vi "CRYAna TSR.vi"(0 "Response":dbl[](array[numeric]) format="%.2f", 1 "Abs/Rel":u16(ring) items=["Absolute", "Relative"], 2 "dz(Hz)":dbl=10.0, 3 "EQ information":T2={"Stimulus EQ Curve"={"Name"="", "Curve"=[], "X data"=1, "Y data"=1, "Z data"=1, "X axis"=0, "Y axis"=1, "Z axis"=1, "X unit"="Hz", "Y unit"="", "Z unit"="deg.", "X dB ref"=1.0, "Y dB ref"=1.0, "Z dB ref"=1.0, "single val"=FALSE, "protected"=FALSE, "display X"=TRUE, "display Y"=TRUE, "display Z"=TRUE, "Test Info"="", "Step No."=0, "Plot Settings"={"Color"=0, "Interpolation"=0, "Point Style"=0, "Line Style"=0, "Point Color"=0, "Line Width"=0, "Bar Plot Style"=0, "Fill To"=0}, "AutoProtect"=FALSE}, "EQ"=FALSE, "EQ Rate"=0.0} {"EQ Rate" format="%.2f"; "Stimulus EQ Curve"."Z data" items=["dB", "Lin"]; "Stimulus EQ Curve"."X data" items=["dB", "Lin"]; "Stimulus EQ Curve"."Y data" items=["dB", "Lin"]; "Stimulus EQ Curve"."Z dB ref" format="%.1f"; "Stimulus EQ Curve"."Z axis" items=["Log", "Lin"]; "Stimulus EQ Curve"."X dB ref" format="%.1f"; "Stimulus EQ Curve"."X axis" items=["Log", "Lin"]; "Stimulus EQ Curve"."Y axis" items=["Log", "Lin"]; "Stimulus EQ Curve"."Y dB ref" format="%.1f"; "Stimulus EQ Curve"."Curve"."z" format="%.2f"; "Stimulus EQ Curve"."Curve"."y" format="%.2f"; "Stimulus EQ Curve"."Curve"."x" format="%.2f"}, 5 "Harmonics":dbl[](array[numeric]) format="%.2f", 7 "Parameter In":T3 {"Over Sample Res" format="%.4f"; "Stop (ms)" format="%.4f"; "Start (ms)" format="%.4f"}, 9 "Resolution":u16=6, 11 "TSR params":T4 {"Sweep Time" format="%.2f"; "Amplit" format="%.2f"; "FStop" format="%.2f"; "FStart" format="%.2f"; "FSamp" format="%.2f"; "Tsamp" format="%.2f"; "NHarm" format="%.2f"; "MStart" format="%.2f"; "MStop" format="%.2f"; "NOffset" format="%.2f"}, 12 "Stimulus":dbl[](array[numeric]) format="%.2f", 15 "Impulse data type(db/Lin)":i32(ring) items=["dB", "Lin"]) -> (4 "Freq resp curves":cluster{cluster{"x":dbl, "y":dbl, "z":dbl}[]}[](array[cluster]) {"?"."z" format="%.2f"; "?"."y" format="%.2f"; "?"."x" format="%.2f"}, 8 "X axis, fundamental":dbl[](array[numeric]) format="%.2f", 10 "Total Noise":dbl[](array[numeric]), 13 "Impulse response":dbl[][](array[numeric]) format="%.2f", 14 "Impulse time axis":dbl[](array[numeric]) format="%.6f")   [LabVIEW 2013]
uses:
  Typedef Control/CRYData Cluster.ctl
  <vilib>/Analysis/NI_AALPro.lvlib
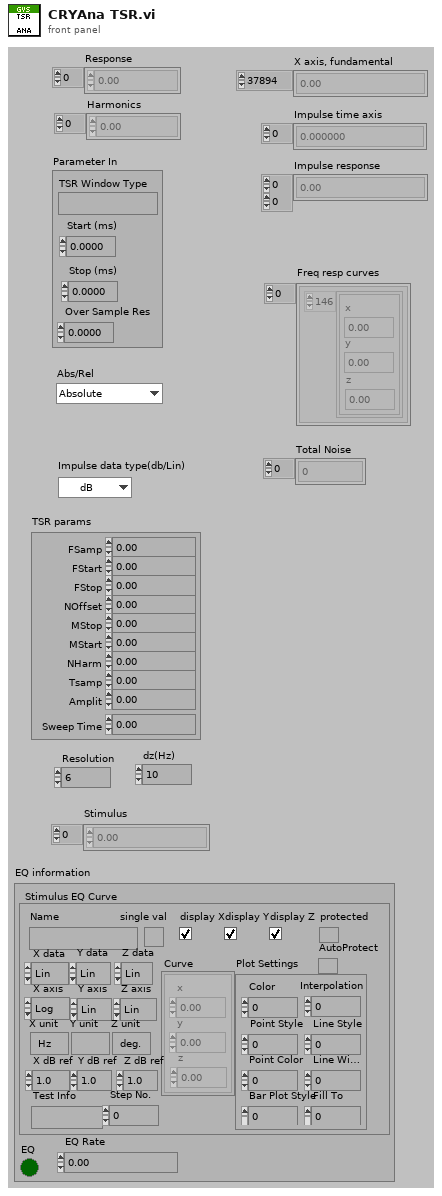
[diagram p1: front panel]
types:
  T1 = typedef "CRYData Cluster.ctl" = cluster{"Name":string, "Curve":cluster{"x":dbl, "y":dbl, "z":dbl}[], "X data":u16, "Y data":u16, "Z data":u16, "X axis":u16, "Y axis":u16, "Z axis":u16, "X unit":string, "Y unit":string, "Z unit":string, "X dB ref":dbl, "Y dB ref":dbl, "Z dB ref":dbl, "single val":bool, "protected":bool, "display X":bool, "display Y":bool, "display Z":bool, "Test Info":string, "Step No.":i32, "Plot Settings":cluster{"Color":u32, "Interpolation":u8, "Point Style":u8, "Line Style":u8, "Point Color":u32, "Line Width":u8, "Bar Plot Style":u8, "Fill To":i16}, "AutoProtect":bool}
  T2 = cluster{"Stimulus EQ Curve":T1, "EQ":bool, "EQ Rate":dbl}
  T3 = cluster{"TSR Window Type":string, "Start (ms)":dbl, "Stop (ms)":dbl, "Over Sample Res":dbl}
  T4 = cluster{"FSamp":dbl, "FStart":dbl, "FStop":dbl, "NOffset":dbl, "MStop":dbl, "MStart":dbl, "NHarm":dbl, "Tsamp":dbl, "Amplit":dbl, "Sweep Time":dbl}
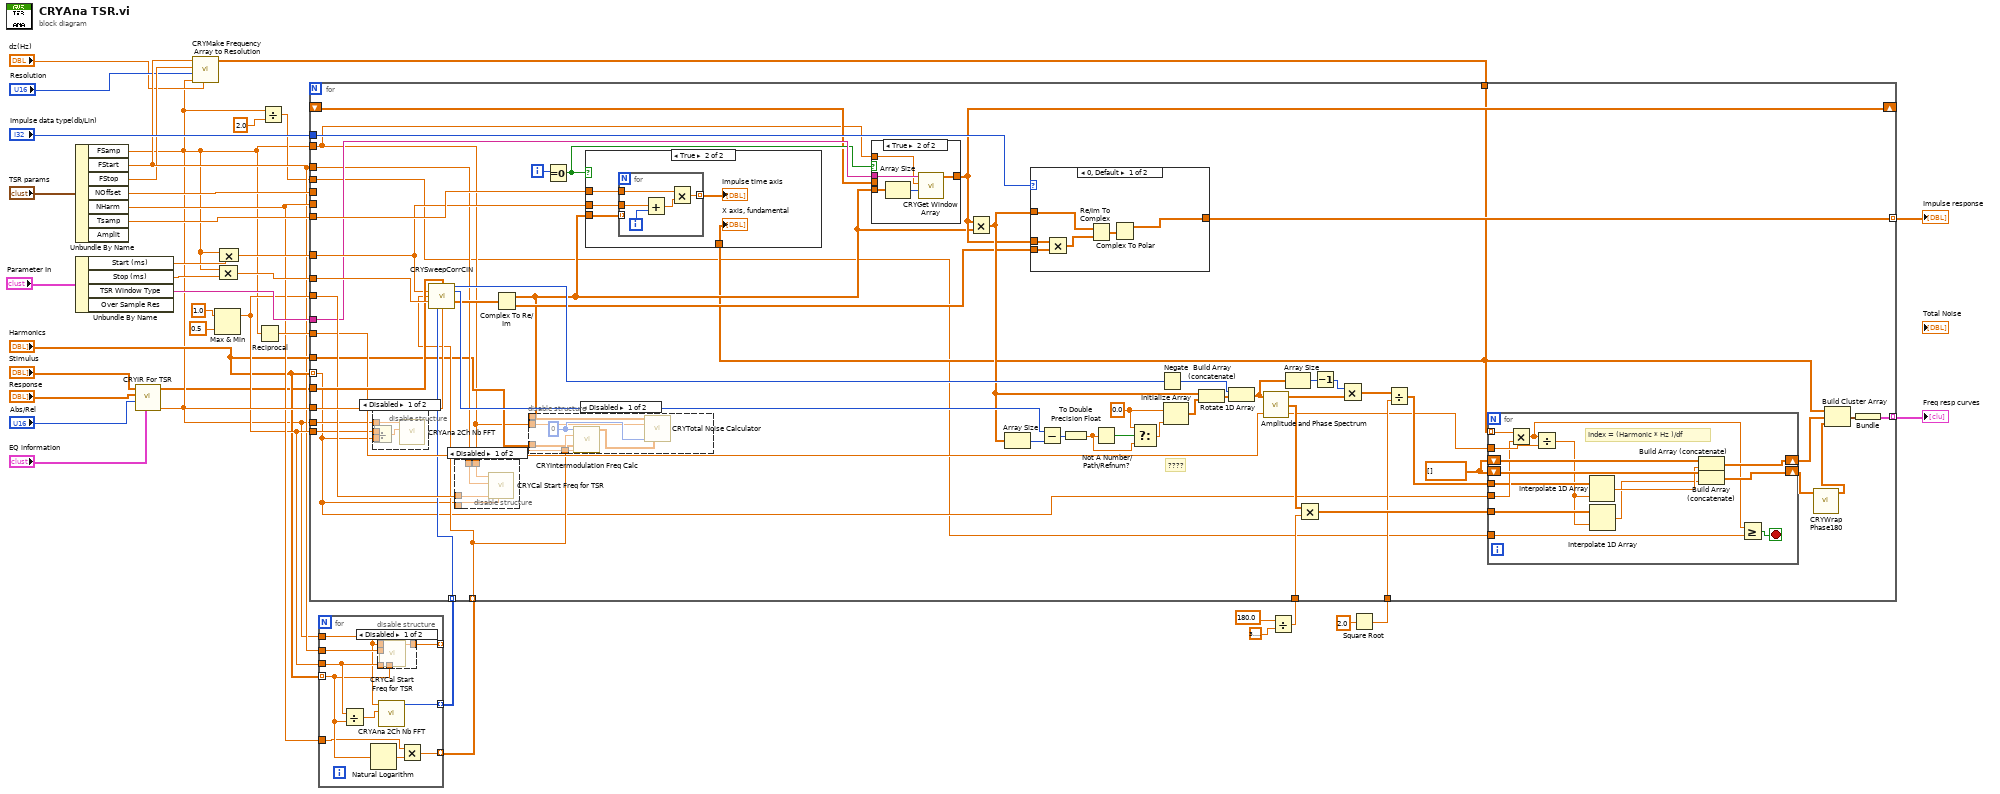
[diagram p0: block diagram]
diagram:
  n1 = Unbundle By Name("TSR params") -> ("FSamp"=w5:dbl, "FStart"=w12:dbl, "FStop"=w11:dbl, "NOffset"=w27:dbl, "NHarm"=w19:dbl, "Tsamp"=w39:dbl)  [unwired: 1 out]
  n2 = Unbundle By Name("Parameter In") -> ("Start (ms)"=w30:dbl, "Stop (ms)"=w29:dbl, "TSR Window Type"=w28:string)  [unwired: 1 out]
  n3 = call "CRYIR For TSR.vi"("EQ information"="EQ information", "Fs"=w5, "Abs/Rel"="Abs/Rel", "Response[y(t)]"="Response", "Stimulus[x(t)]"="Stimulus") -> ("T0"=w26:dbl, "Deconvolved Response"=w4:cdb[])  [unwired: 2 in, 3 out]
  n4 = call "CRYMake Frequency Array to Resolution.vi"("dz(Hz)"="dz(Hz)", "Fs"=w5, "Resolution"="Resolution", "Stop Freq"=w11, "Start Freq"=w12) -> ("Frequency Array"=w8:dbl[])  [unwired: 6 in]
  n5 = Max & Min(x=1.0, y=0.5) -> (max(x,y)=w14:dbl)  [unwired: 1 out]
  n6 = Compound Arithmetic op=MULTIPLY(w5, w29) -> (w33:dbl)
  n7 = Compound Arithmetic op=MULTIPLY(w5, w30) -> (w32:dbl)
  n8 = Reciprocal(x=w5) -> (1/x=w25:dbl)
  n9 = Divide(x=w5, y=2.0) -> (x/y=w6:dbl)
  n10 = for {
    tunnel: "Harmonics" -> [w42] mode=indexing
    tunnel: w14 -> [w46]
    tunnel: w12 -> [w49]
    tunnel: w5 -> [w45]
    tunnel: [w48] -> _ mode=indexing
    tunnel: [w44] -> w20 mode=indexing
    tunnel: w19 -> [w41]
    tunnel: [w40] -> w18 mode=indexing
    n11 = Divide(x=w46, y=w42) -> (x/y=w47:dbl)
    n12 = Natural Logarithm(1:w42) -> (0:w43:dbl)
    n13 = disable-structure shown="Disabled" {
      disable-tunnel: w49 -> [w54 _]
      disable-tunnel: [w53 _] -> w48
      disable-tunnel: w46 -> [w52 _]
      disable-tunnel: w45 -> [w51 _]
      disable-tunnel: w42 -> [w50 _]
      frame Disabled {
        n14 = call "CRYCal Start Freq for TSR.vi"("Hn"=w50, "Over-samples Res."=w52, "FStart"=w54, "Fs"=w51) -> ("Start Fs"=w53:dbl)  [unwired: 6 in, 1 out]
      }
      frame Enabled {
      }
    }
    n15 = call "CRYAna 2Ch Nb FFT.vi"("dF(Hz)"=w47, "Fs(Hz)"=w45) -> ("FFT Size(Sp)"=w44:i32)  [unwired: 6 in, 3 out]
    n16 = Multiply(x=w41, y=w43) -> (x*y=w40:dbl)
  }
  n17 = Divide(x=180.0, y=3.141592653589793) -> (x/y=w36:dbl)
  n18 = Square Root(x=2.0 ("element")) -> (sqrt(x)=w2:dbl)
  n19 = for {
    tunnel: "Harmonics" -> [w58] mode=indexing
    tunnel: [w85] -> w22 mode=indexing
    tunnel: w5 -> [w61]
    tunnel: w12 -> [w82]
    tunnel: w6 -> [w57]
    tunnel: w27 -> [_]
    tunnel: w19 -> [_]
    tunnel: w39 -> [w110]
    tunnel: w36 -> [w107]
    tunnel: "Impulse data type(db/Lin)" -> [w87]
    tunnel: w32 -> [w101]
    tunnel: w33 -> [w109]
    tunnel: w28 -> [w90]
    tunnel: w4 -> [w104]
    tunnel: [w108] -> w21 mode=indexing
    tunnel: w14 -> [w103]
    tunnel: w26 -> [w105]
    tunnel: w25 -> [w91]
    tunnel: w5 -> [w89]
    tunnel: w14 -> [w88]
    tunnel: w20 -> [w76] mode=indexing
    tunnel: w18 -> [w63] mode=indexing
    shift-right: [w72] -> _
    shift-left: _ -> [w71]
    tunnel: w2 -> [w70]
    tunnel: "Harmonics" -> [w62]
    tunnel: w8 -> [w60]
    i -> [w83]
    w68 = 0.0 ("element")
    w81 = dbl[] []
    # "????"
    n20 = disable-structure shown="Disabled" {
      disable-tunnel: w89 -> [w126 _]
      disable-tunnel: w88 -> [w124 _]
      disable-tunnel: w58 -> [w123 _]
      frame Disabled {
        n21 = Divide(x=w124, y=w123) -> (x/y=w125:dbl)
        n22 = call "CRYAna 2Ch Nb FFT.vi"("dF(Hz)"=w125, "Fs(Hz)"=w126) -> ()  [unwired: 6 in, 4 out]
      }
      frame Enabled {
      }
    }
    n23 = call "CRYSweepCorrCIN.vi"("Deconv Response"=w104, "MStart"=w101, "NHarm"=w63, "MStop"=w109, "FFT size"=w76, "T0"=w105) -> ("T0 Position"=w93:i32, "FFT Size"=w94:i32, "Impulse Response"=w92:cdb[])  [unwired: 7 in]
    n24 = disable-structure shown="Disabled" {
      disable-tunnel: w103 -> [w130 _]
      disable-tunnel: w61 -> [w129 _]
      disable-tunnel: w82 -> [w128 _]
      disable-tunnel: w58 -> [w127 _]
      frame Disabled {
        n25 = call "CRYCal Start Freq for TSR.vi"("Hn"=w127, "Over-samples Res."=w130, "FStart"=w128, "Fs"=w129) -> ()  [unwired: 6 in, 2 out]
      }
      frame Enabled {
      }
    }
    n26 = Complex To Re/Im(x + iy=w92) -> (x=w64:dbl[], y=w74:dbl[])
    n27 = disable-structure shown="Disabled" {
      disable-tunnel: w64 -> [w116 _]
      disable-tunnel: w63 -> [w113 _]
      disable-tunnel: w62 -> [w112 _]
      disable-tunnel: w61 -> [w111 _]
      frame Disabled {
        w115 = u16 0 ("Type")
        n28 = call "CRYIntermodulation Freq Calc.vi"("Type"=w115, "Freq1 In"=w113, "Orders"=w112, "Fs"=w111) -> ("Frequency Array Out"=w114:dbl[])  [unwired: 11 in]
        n29 = call "CRYTotal Noise Calculator.vi"("Input Signal"=w116, "Fs"=w111, "Type(Harm,Inter,Diff)"=w115, "Freq Array"=w114) -> ()  [unwired: 10 in, 2 out]
      }
      frame Enabled {
      }
    }
    n30 = Equal To 0?(x=w83) -> (x = 0?=w73:bool)
    n31 = case shown="True" w73 {
      tunnel: w110 -> [_ w157]
      tunnel: w101 -> [_ w156]
      tunnel: w64 -> [_ w155]
      tunnel: w60 -> [_ w153]
      frame False {
      }
      frame True {
        n32 = for {
          tunnel: [w161] -> w154 mode=indexing
          tunnel: w156 -> [w159]
          tunnel: w157 -> [w158]
          tunnel: w155 -> [_] mode=indexing
          i -> [w162]
          n33 = Add(x=w159, y=w162) -> (x+y=w160:dbl)
          n34 = Multiply(x=w158, y=w160) -> (x*y=w161:dbl)
        }
        "Impulse time axis" <- w154
        "X axis, fundamental" <- w153
      }
    }
    n35 = case shown="True" w73 {
      tunnel: w90 -> [_ w122]
      tunnel: w61 -> [_ w121]
      tunnel: w64 -> [_ w119]
      tunnel: [w117 w118] -> w72
      tunnel: w71 -> [w117 _]
      frame False {
      }
      frame True {
        n36 = Array Size(array=w119) -> (size(s)=w120:i32)
        n37 = call "CRYGet Window Array.vi"("size(s)"=w120, "Fs"=w121, "TSR Window Name"=w122) -> ("Window Array"=w118:dbl[])  [unwired: 8 in]
      }
    }
    n38 = Multiply(x=w72, y=w64) -> (x*y=w86:dbl[])
    n39 = Array Size(array=w86) -> (size(s)=w95:i32)
    n40 = case shown="0, Default" w87 {
      tunnel: w86 -> [w136 w137]
      tunnel: [w134 w137] -> w85
      tunnel: w72 -> [w133 _]
      tunnel: w74 -> [w131 _]
      frame 0, Default {
        n41 = Multiply(x=w133, y=w131) -> (x*y=w132:dbl[])
        n42 = Re/Im To Complex(1:w132, 2:w136) -> (0:w135:cdb[])
        n43 = Complex To Polar(r * e^(i*theta)=w135) -> (r=w134:dbl[])  [unwired: 1 out]
      }
      frame 1 {
      }
    }
    n44 = Subtract(x=w94, y=w95) -> (x-y=w67:i32)
    n45 = To Double Precision Float(number=w67) -> (double precision float=w65:dbl)
    n46 = Not A Number/Path/Refnum?(number/path/refnum=w65) -> (NaN/Path/Refnum?=w69:bool)
    n47 = Select(t=w68, s=w69, f=w65) -> (s? t:f=w66:dbl)
    n48 = Negate(x=w93) -> (-x=w98:i32)
    n49 = Initialize Array(w68, w66) -> (w96:dbl[])
    n50 = Build Array (concatenate)(w86, w96) -> (w97:dbl[])
    n51 = Rotate 1D Array(1:w97, 2:w98) -> (0:w84:dbl[])
    n52 = call <vilib>:"Amplitude and Phase Spectrum.vi"("dt"=w91, "Signal (V)"=w84) -> ("df"=w59:dbl, "Amp Spectrum Phase (radians)"=w106:dbl[], "Amp Spectrum Mag (Vrms)"=w78:dbl[])  [unwired: 1 in]
    n53 = Array Size(array=w84) -> (size(s)=w100:i32)
    n54 = Multiply(x=w106, y=w107) -> (x*y=w79:dbl[])
    n55 = Decrement(x=w100) -> (x-1=w77:i32)
    n56 = Multiply(x=w77, y=w78) -> (x*y=w75:dbl[])
    n57 = Divide(x=w75, y=w70) -> (x/y=w80:dbl[])
    n58 = for {
      tunnel: w80 -> [w142]
      tunnel: w79 -> [w141]
      shift-right: [w151] -> w99
      shift-left: w81 -> [w152]
      shift-right: [w149] -> w56
      shift-left: w81 -> [w150]
      tunnel: w60 -> [w147] mode=indexing
      tunnel: w59 -> [w148]
      tunnel: w58 -> [w146]
      tunnel: w57 -> [w143]
      stop <- w145 stop-if-true
      # "Index = (Harmonic * Hz )/df"
      n59 = Multiply(x=w147, y=w146) -> (x*y=w144:dbl)
      n60 = Divide(x=w144, y=w148) -> (x/y=w140:dbl)
      n61 = Interpolate 1D Array(1:w140, 2:w142) -> (0:w139:dbl)
      n62 = Interpolate 1D Array(1:w140, 2:w141) -> (0:w138:dbl)
      n63 = Build Array (concatenate)(w152, w139) -> (w151:dbl[])
      n64 = Build Array (concatenate)(w150, w138) -> (w149:dbl[])
      n65 = Greater Or Equal?(x=w144, y=w143) -> (x >= y?=w145:bool)
    }
    n66 = call "CRYWrap Phase180.vi"("Phase In"=w56) -> ("Phase Out"=w55:dbl[])  [unwired: 10 in]
    n67 = Build Cluster Array(w60, w99, w55) -> (w102:cluster{dbl, dbl, "Phase In":dbl}[])
    n68 = Bundle(w102) -> (w108:cluster{cluster{dbl, dbl, "Phase In":dbl}[]})  [unwired: 1 in]
  }
  "Impulse response" <- w22
  "Freq resp curves" <- w21
